vi "For Range.vi"   [LabVIEW 2018]
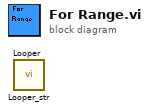
[diagram p0: block diagram]
diagram:
  n1 = call "Looper_str.vi"() -> ()  [unwired: 10 in, 2 out]
  n2 = call "Looper.vi"() -> ()  [unwired: 10 in, 2 out]
